vi "Configure Modulation (Digital).vi"(0 "VISA resource name":refnum<visa-resource-name>, 1 "Enable Digital Modulation (T:Enable)":bool=TRUE, 2 "Modulation Type (6: pi/4 DQPSK)":u16(ring)=6 items=["BPSK", "QPSK", "IS-95 QPSK", "Gray Coded QPSK", "OQPSK", "IS-95 OQPSK", "pi/4 DQPSK", "8PSK", "16PSK", "D8PSK", "MSK", "2-Lvl FSK", "4-Lvl FSK", "8-Lvl FSK", "16-Lvl FSK", "C4FM", "4QAM", "16QAM", "32QAM", "64QAM", "128QAM", "256QAM", "User I/Q", "User FSK", "ASK", "UQPSK", "EDGE", "1024QAM", "VSA 16QAM", "VSA 32QAM", "VSA 64QAM", "VSA 128QAM", "VSA 256QAM", "VSA 512QAM", "VSA 1024QAM"], 3 "FSK Frequency Deviation (400 Hz)":dbl=400.0, 5 "Multicarrier Phase (0: Fixed)":u16(ring) items=["Fixed", "Random"], 7 "Standard (1: NADC)":u16(ring)=1 items=["GSM", "NADC", "PDC", "PHS", "DECT", "APCO 25 w/C4FM", "APCO w/CQPSK", "CDPD", "PWT", "EDGE", "TETRA", "Multicarrier", "Select File", "Bluetooth", "Default"], 9 "File Name (\"\")":string, 11 "error in (no error)":errorcluster, 12 "Symbol Rate (24.3 ksps)":dbl=24300.0, 13 "ASK Depth (100 percent)":dbl=100.0) -> (4 "VISA resource name out":refnum<visa-resource-name>, 15 "error out":errorcluster)   [LabVIEW 2018, in "Agilent PSG MXG Series.lvlib"]
doc: "Configures the state, modulation type, standard and symbol rate for the digital modulation.\n\n<B>Notes:</B>\n(1) This VI is valid only in E8267C, E8267D, N5162A, N5182A, N5172B, N5182B.\n\n(2) For E8267C, this VI is valid only when the instrument installs <B>Option 002</B> (Internal baseband generator) or <B>Option 602</B> (Digital bus baseband generator).\n\n(3) For E8267D, this VI is valid only when the instrument installs <B>Option 601</B> or <B>Option 602</B> (Internal baseband generator).\n\n(4) For N5162A and N5182A, this VI is valid only when the instrument installs <B>Option 651</B> or <B>Option 652</B> or <B>Option 654</B> (Internal baseband generator).\n\n(5) For N5172B and N5182B, this VI is valid only when the instrument installs <B>Option 431</B>."
uses:
  Agilent PSG MXG Series.lvlib
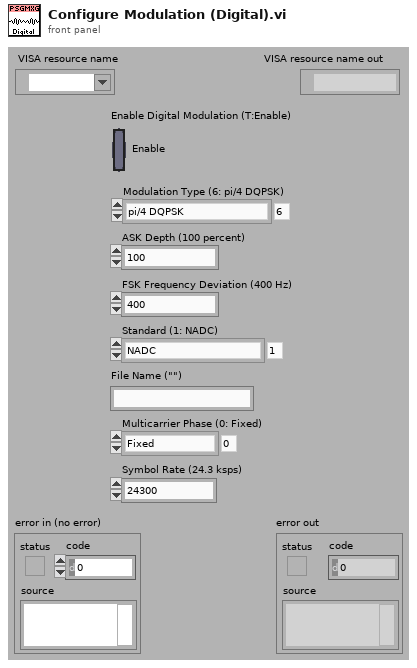
[diagram p1: front panel]
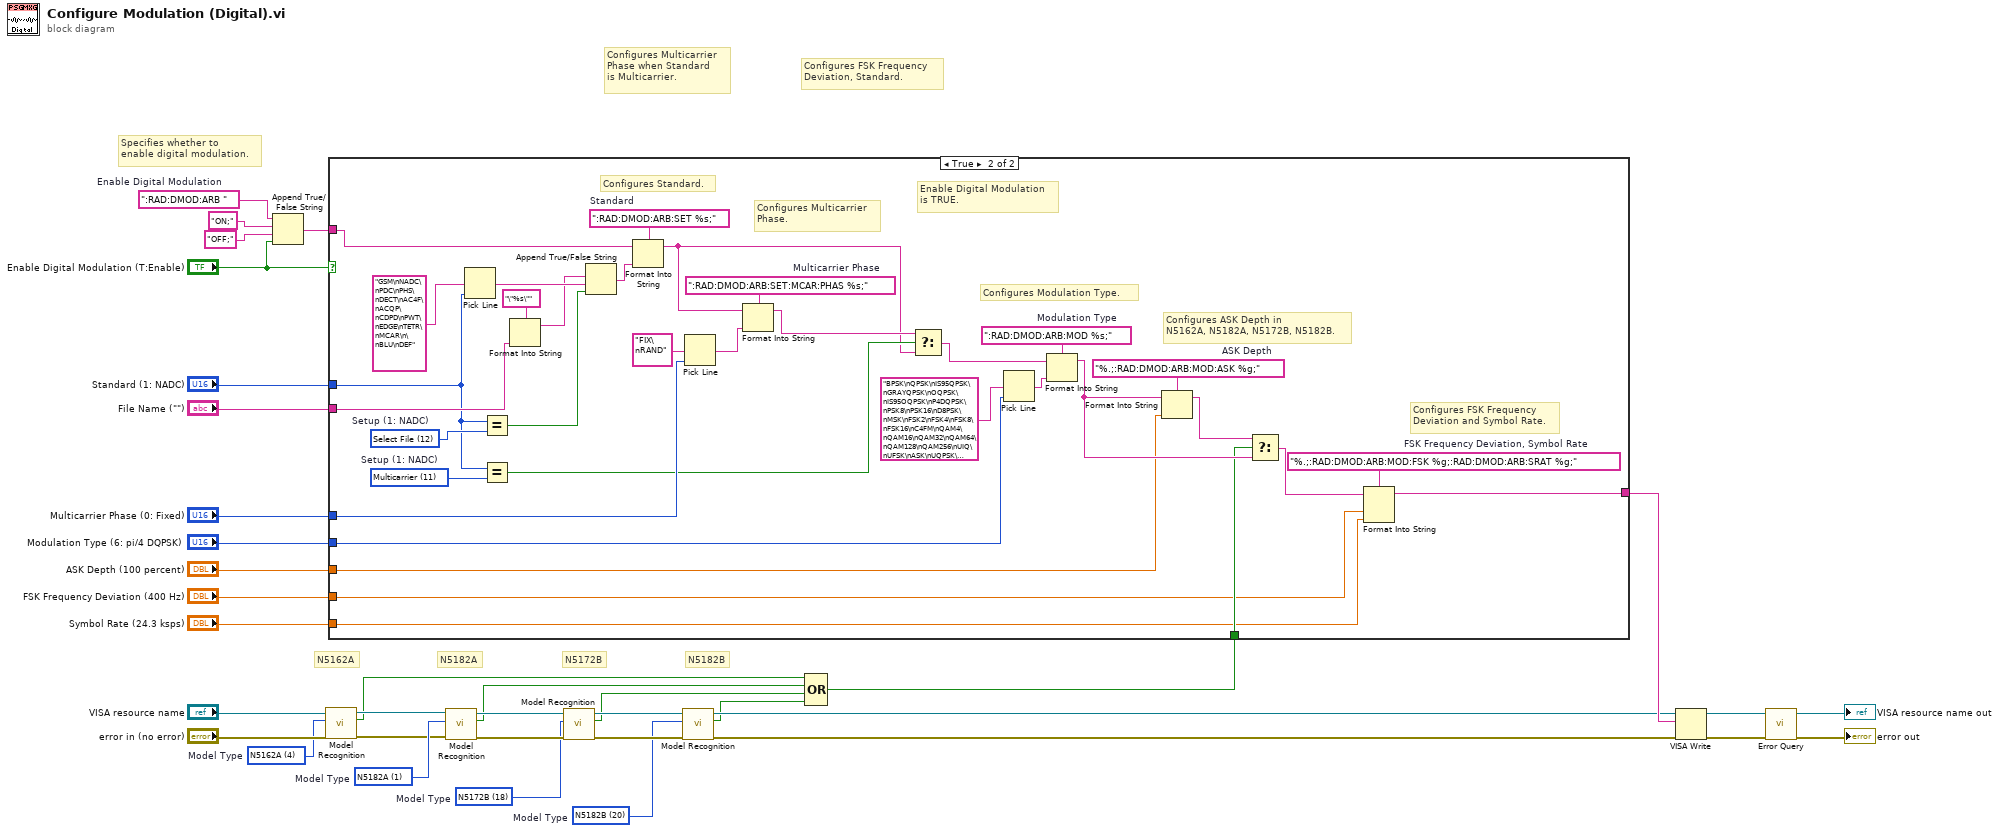
[diagram p0: block diagram]
diagram:
  w2 = u16 4 items=["N5181A"=0, "N5182A"=1, "N5183A"=2, "N5161A"=3, "N5162A"=4, "E8241A"=5, "E8244A"=6, "E8251A"=7, "E8254A"=8, "E8247C"=10, "E8257C"=11, "E8267C"=12, "E8257D"=15, "E8267D"=16, "N5171B"=17, "N5172B"=18, "N5181B"=19, "N5182B"=20]  # Model Type
  w11 = u16 20 items=["N5181A"=0, "N5182A"=1, "N5183A"=2, "N5161A"=3, "N5162A"=4, "E8241A"=5, "E8244A"=6, "E8251A"=7, "E8254A"=8, "E8247C"=10, "E8257C"=11, "E8267C"=12, "E8257D"=15, "E8267D"=16, "N5171B"=17, "N5172B"=18, "N5181B"=19, "N5182B"=20]  # Model Type
  w12 = u16 18 items=["N5181A"=0, "N5182A"=1, "N5183A"=2, "N5161A"=3, "N5162A"=4, "E8241A"=5, "E8244A"=6, "E8251A"=7, "E8254A"=8, "E8247C"=10, "E8257C"=11, "E8267C"=12, "E8257D"=15, "E8267D"=16, "N5171B"=17, "N5172B"=18, "N5181B"=19, "N5182B"=20]  # Model Type
  w19 = u16 1 items=["N5181A"=0, "N5182A"=1, "N5183A"=2, "N5161A"=3, "N5162A"=4, "E8241A"=5, "E8244A"=6, "E8251A"=7, "E8254A"=8, "E8247C"=10, "E8257C"=11, "E8267C"=12, "E8257D"=15, "E8267D"=16, "N5171B"=17, "N5172B"=18, "N5181B"=19, "N5182B"=20]  # Model Type
  w36 = ":RAD:DMOD:ARB "  # Enable Digital Modulation
  # "N5162A"
  # "N5182B"
  # "N5172B"
  # "Configures Multicarrier\nPhase when Standard\nis Multicarrier."
  # "Configures FSK Frequency\nDeviation, Standard."
  # "Specifies whether to\nenable digital modulation."
  # "N5182A"
  n1 = Append True/False String(1:"Enable Digital Modulation (T:Enable)", 2:"OFF;" ("false string"), 3:"ON;" ("true string"), 4:w36) -> (0:w32:string)
  n2 = call "Model Recognition.vi"("error in (no error)"="error in (no error)", "Model Type (0: N5181A)"=w2, "VISA resource name"="VISA resource name") -> ("error out"=w5:errorcluster, "Is Model Correct"=w1:bool, "VISA resource name out"=w3:refnum<visa-resource-name>)  [unwired: 6 out]
  n3 = call "Model Recognition.vi"("error in (no error)"=w5, "Model Type (0: N5181A)"=w19, "VISA resource name"=w3) -> ("error out"=w16:errorcluster, "Is Model Correct"=w8:bool, "VISA resource name out"=w18:refnum<visa-resource-name>)  [unwired: 6 out]
  n4 = call "Model Recognition.vi"("error in (no error)"=w16, "Model Type (0: N5181A)"=w12, "VISA resource name"=w18) -> ("error out"=w15:errorcluster, "Is Model Correct"=w9:bool, "VISA resource name out"=w17:refnum<visa-resource-name>)  [unwired: 6 out]
  n5 = call "Model Recognition.vi"("error in (no error)"=w15, "Model Type (0: N5181A)"=w11, "VISA resource name"=w17) -> ("error out"=w13:errorcluster, "Is Model Correct"=w10:bool, "VISA resource name out"=w14:refnum<visa-resource-name>)  [unwired: 6 out]
  n6 = Compound Arithmetic op=OR(w1, w8, w9, w10) -> (w7:bool)
  n7 = case shown="True" "Enable Digital Modulation (T:Enable)" {
    tunnel: w32 -> [w37 w55]
    tunnel: "Modulation Type (6: pi/4 DQPSK)" -> [_ w42]
    tunnel: "FSK Frequency Deviation (400 Hz)" -> [_ w40]
    tunnel: "Standard (1: NADC)" -> [_ w60]
    tunnel: "File Name (\"\")" -> [_ w66]
    tunnel: "Multicarrier Phase (0: Fixed)" -> [_ w61]
    tunnel: "Symbol Rate (24.3 ksps)" -> [_ w39]
    tunnel: [w37 w56] -> w25
    tunnel: "ASK Depth (100 percent)" -> [_ w41]
    tunnel: w7 -> [_ w45]
    frame False {
      # "Enable Digital Modulation\nis FALSE."
    }
    frame True {
      w44 = "%.;:RAD:DMOD:ARB:MOD:FSK %g;:RAD:DMOD:ARB:SRAT %g;"  # FSK Frequency Deviation, Symbol Rate
      w49 = "%.;:RAD:DMOD:ARB:MOD:ASK %g;"  # ASK Depth
      w47 = ":RAD:DMOD:ARB:MOD %s;"  # Modulation Type
      w54 = ":RAD:DMOD:ARB:SET %s;"  # Standard
      w59 = u16 11 items=["GSM", "NADC", "PDC", "PHS", "DECT", "APCO 25 w/C4FM", "APCO w/CQPSK", "CDPD", "PWT", "EDGE", "TETRA", "Multicarrier", "Select File"]  # Setup (1: NADC)
      w64 = ":RAD:DMOD:ARB:SET:MCAR:PHAS %s;"  # Multicarrier Phase
      w70 = u16 12 items=["GSM", "NADC", "PDC", "PHS", "DECT", "APCO 25 w/C4FM", "APCO w/CQPSK", "CDPD", "PWT", "EDGE", "TETRA", "Multicarrier", "Select File"]  # Setup (1: NADC)
      # "Configures Multicarrier\nPhase."
      # "Configures Standard."
      # "Configures ASK Depth in\nN5162A, N5182A, N5172B, N5182B."
      # "Configures Modulation Type."
      # "Configures FSK Frequency\nDeviation and Symbol Rate."
      # "Enable Digital Modulation\nis TRUE."
      n8 = Pick Line(multi-line string="GSM\nNADC\nPDC\nPHS\nDECT\nAC4F\nACQP\nCDPD\nPWT\nEDGE\nTETR\nMCAR\n\nBLU\nDEF", line index=w60) -> (output string=w68:string)  [unwired: 1 out]
      n9 = Equal?(x=w60, y=w70) -> (x = y?=w69:bool)
      n10 = Equal?(x=w60, y=w59) -> (x = y?=w57:bool)
      n11 = Format Into String(format string="\"%s\"", w66) -> (resulting string=w65:string)  [unwired: 2 in, 1 out]
      n12 = Append True/False String(1:w69, 2:w68, 3:w65) -> (0:w53:string)  [unwired: 1 out]
      n13 = Format Into String(format string=w54, initial string=w55, w53) -> (resulting string=w52:string)  [unwired: 1 in, 1 out]
      n14 = Pick Line(multi-line string="FIX\nRAND", line index=w61) -> (output string=w63:string)  [unwired: 1 out]
      n15 = Format Into String(format string=w64, initial string=w52, w63) -> (resulting string=w58:string)  [unwired: 1 in, 1 out]
      n16 = Select(t=w58, s=w57, f=w52) -> (s? t:f=w46:string)
      n17 = Pick Line(multi-line string="BPSK\nQPSK\nIS95QPSK\nGRAYQPSK\nOQPSK\nIS95OQPSK\nP4DQPSK\nPSK8\nPSK16\nD8PSK\nMSK\nFSK2\nFSK4\nFSK8\nFSK16\nC4FM\nQAM4\nQAM16\nQAM32\nQAM64\nQAM128\nQAM256\nUIQ\nUFSK\nASK\nUQPSK\nEDGE\nQAM1024\nVSAQAM16\nVSAQAM32\nVSAQAM64\nVSAQAM128\nVSAQAM256\nVSAQAM512\nVSAQAM1024", line index=w42) -> (output string=w48:string)  [unwired: 1 out]
      n18 = Format Into String(format string=w47, initial string=w46, w48) -> (resulting string=w51:string)  [unwired: 1 in, 1 out]
      n19 = Format Into String(format string=w49, initial string=w51, w41) -> (resulting string=w50:string)  [unwired: 1 in, 1 out]
      n20 = Select(t=w50, s=w45, f=w51) -> (s? t:f=w43:string)
      n21 = Format Into String(format string=w44, initial string=w43, w40, w39) -> (resulting string=w56:string)  [unwired: 1 in, 1 out]
    }
  }
  n22 = VISA Write(VISA resource name=w14, write buffer=w25, error in (no error)=w13) -> (VISA resource name out=w24:refnum<visa-resource-name>, error out=w23:errorcluster)  [unwired: 1 out]
  n23 = call "Error Query.vi"("error in (no error)"=w23, "VISA resource name"=w24) -> ("error out"=→"error out":errorcluster, "VISA resource name out"=→"VISA resource name out":refnum<visa-resource-name>)  [unwired: 8 out]
